vi "RTS Power Select Logic.vi"(8 "Error In":errorcluster, 10 "Voltage in":dbl, 11 "Frequency":T2 items=["60 Hz", "50 Hz"]) -> (0 "Error Out":errorcluster, 1 "Voltage Range Selector 1":T1, 3 "Voltage out":dbl)   [LabVIEW 2018]
uses:
  Type Definitions/RTS Frequency Selector.ctl
  Drivers/WAGO 750-881/Type Definitions/Wago Voltage Range Selector.ctl
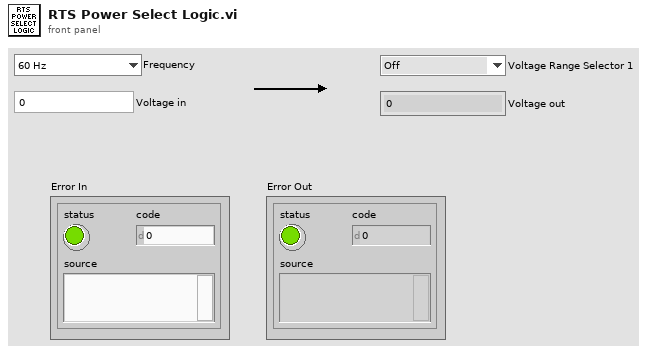
[diagram p1: front panel]
types:
  T1 = typedef "Wago Voltage Range Selector.ctl" = enum16{"Off", "115V 60Hz", "230V 60Hz", "100V 50Hz", "230V 50Hz"}
  T2 = typedef "RTS Frequency Selector.ctl" = u16
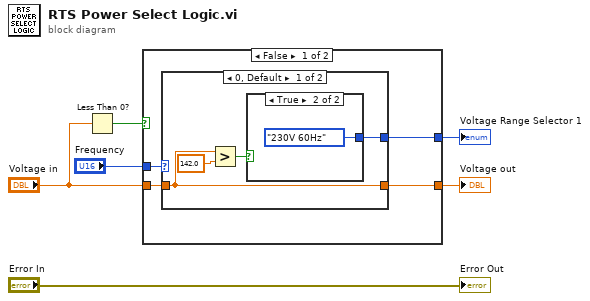
[diagram p0: block diagram]
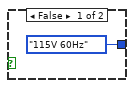
[diagram p2: hidden frame]
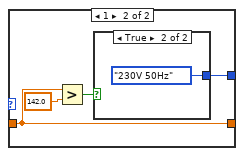
[diagram p3: hidden frame]
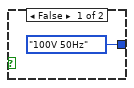
[diagram p4: hidden frame]
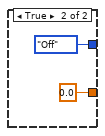
[diagram p5: hidden frame]
diagram:
  n1 = Less Than 0?(x="Voltage in") -> (x < 0?=w4:bool)
  n2 = case shown="False" w4 {
    tunnel: "Frequency" -> [w10 _]
    tunnel: "Voltage in" -> [w9 _]
    tunnel: [w8 Wago_Voltage_Range_Selector."Off" ("Voltage Range Selector 1")] -> w6
    tunnel: [w7 0.0 ("Voltage in")] -> w5
    frame False {
      n3 = case shown="0, Default" w10 {
        tunnel: w9 -> [w11 w17]
        tunnel: [w12 w18] -> w8
        tunnel: [w11 w17] -> w7
        frame 0, Default {
          n4 = Greater?(x=w11, y=142.0) -> (0:w13:bool)
          n5 = case shown="True" w13 {
            tunnel: [Wago_Voltage_Range_Selector."115V 60Hz" ("Voltage Range Selector 1") Wago_Voltage_Range_Selector."230V 60Hz" ("Voltage Range Selector 1")] -> w12
            frame False {
            }
            frame True {
            }
          }
        }
        frame 1 {
          n6 = Greater?(x=w17, y=142.0) -> (0:w19:bool)
          n7 = case shown="True" w19 {
            tunnel: [Wago_Voltage_Range_Selector."100V 50Hz" ("Voltage Range Selector 1") Wago_Voltage_Range_Selector."230V 50Hz" ("Voltage Range Selector 1")] -> w18
            frame False {
            }
            frame True {
            }
          }
        }
      }
    }
    frame True {
    }
  }
  "Voltage Range Selector 1" <- w6
  "Voltage out" <- w5
  "Error Out" <- "Error In"
